vi "Read ADU Packet.vi"(8 "error in":errorcluster, 10 "Network Protocol":refnum<class "Network Protocol.lvclass">, 11 "ASCII transmission data unit in":refnum<class "ASCII Data Unit.lvclass">) -> (0 "error out":errorcluster, 1 "modbus data unit":refnum<class "Modbus Data Unit.lvclass">, 2 "Network Protocol out":refnum<class "Network Protocol.lvclass">, 3 "ASCII transmission data unit out":refnum<class "ASCII Data Unit.lvclass">, 5 "PDU Valid?":bool)   [LabVIEW 2013, in "Modbus Library - Advance.lvlib" / "ASCII Data Unit.lvclass"]
uses:
  ASCII Data Unit.lvclass
  Modbus Data Unit/Modbus Data Unit.lvclass
  Network Protocol/Network Protocol.lvclass
  Network Protocol/Network Master/Serial/Serial Master.lvclass
  Network Protocol/Network Master/Serial/Serial Master.lvclass/Serial Master.ctl
  Network Protocol/Network Slave/Serial/Serial Slave.lvclass
  Network Protocol/Network Slave/Serial/Serial Slave.lvclass/Serial Slave.ctl
  Transmission Data Unit.lvclass/Transmission Data Unit.ctl
  Serial Interface/Serial Data Unit.lvclass/Serial Data Unit.ctl
  Modbus Data Unit/Modbus Data Unit.lvclass/Modbus Data Unit.ctl
  ASCII Data Unit.lvclass/ASCII Data Unit.ctl
  Serial Interface/Serial acquisition states.ctl
  <vilib>/ErrorRing/Error Ring.xnode
  Transmission Data Unit.lvclass
  Serial Interface/Serial Data Unit.lvclass
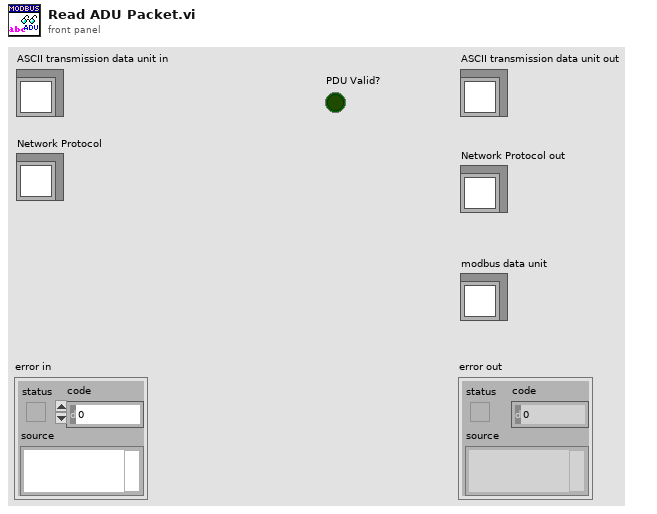
[diagram p1: front panel]
types:
  T1 = typedef "Modbus Library - Advance.lvlib/Serial Data Unit.lvclass/Serial acquisition states.ctl" = enum16{"Wait for frame", "Check for validity"}
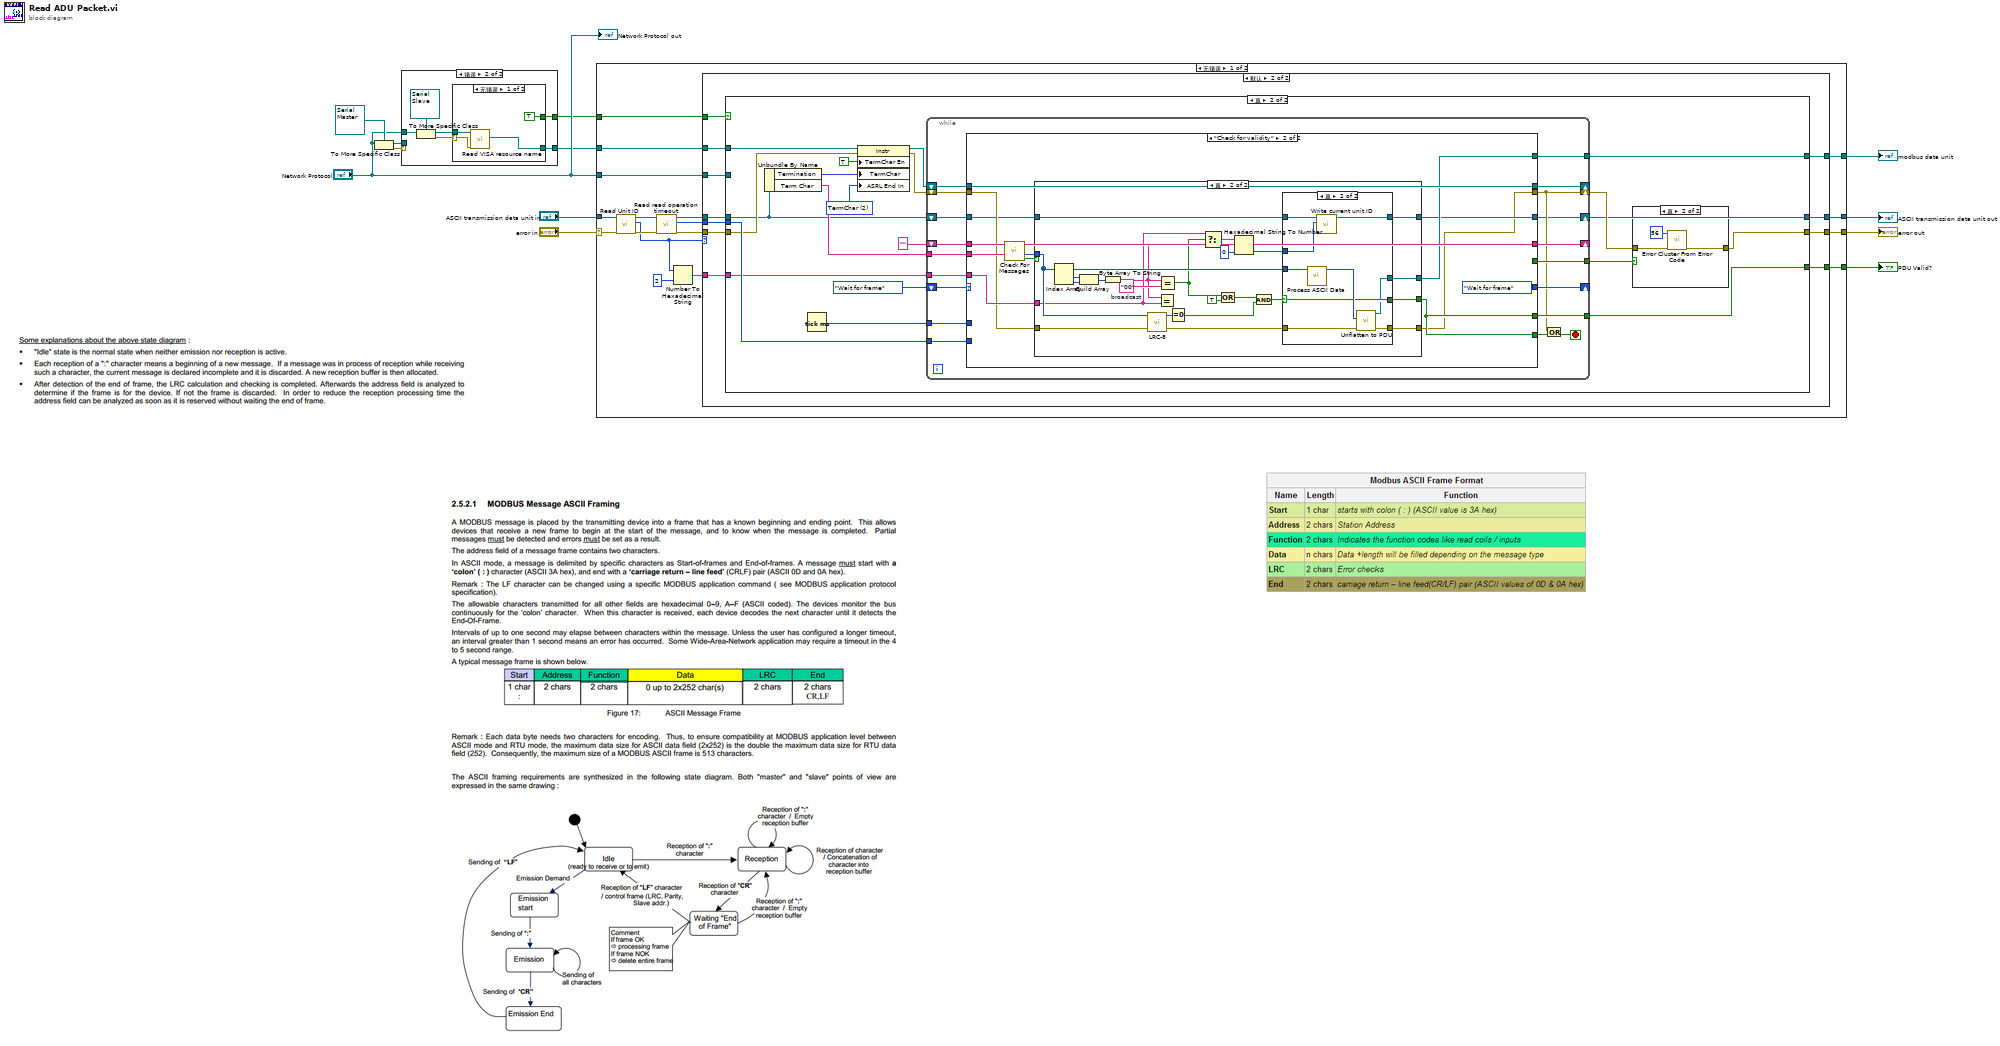
[diagram p0: block diagram]
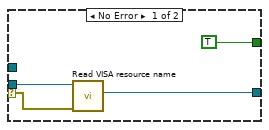
[diagram p2: hidden frame]
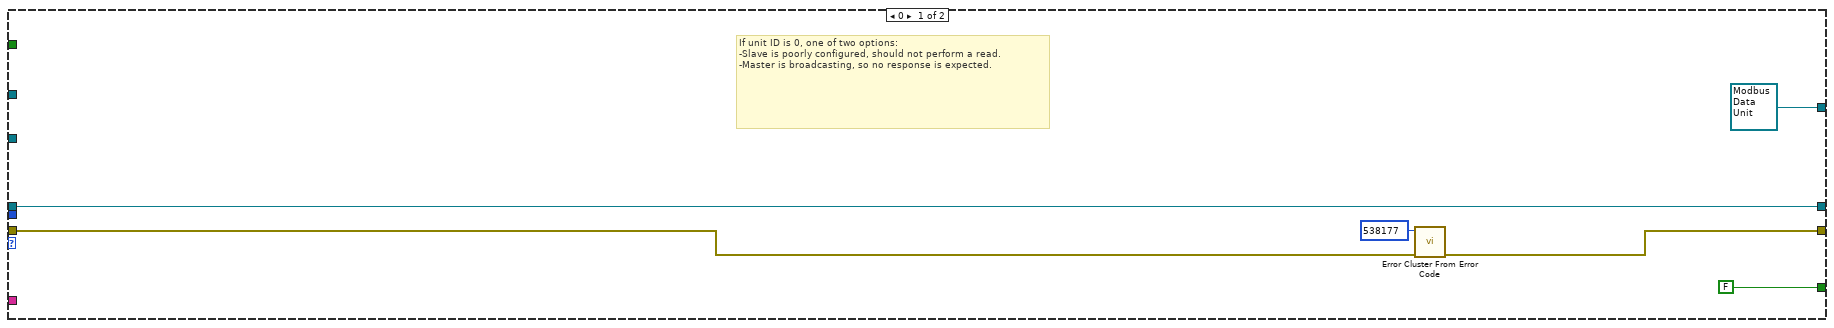
[diagram p4: hidden frame]
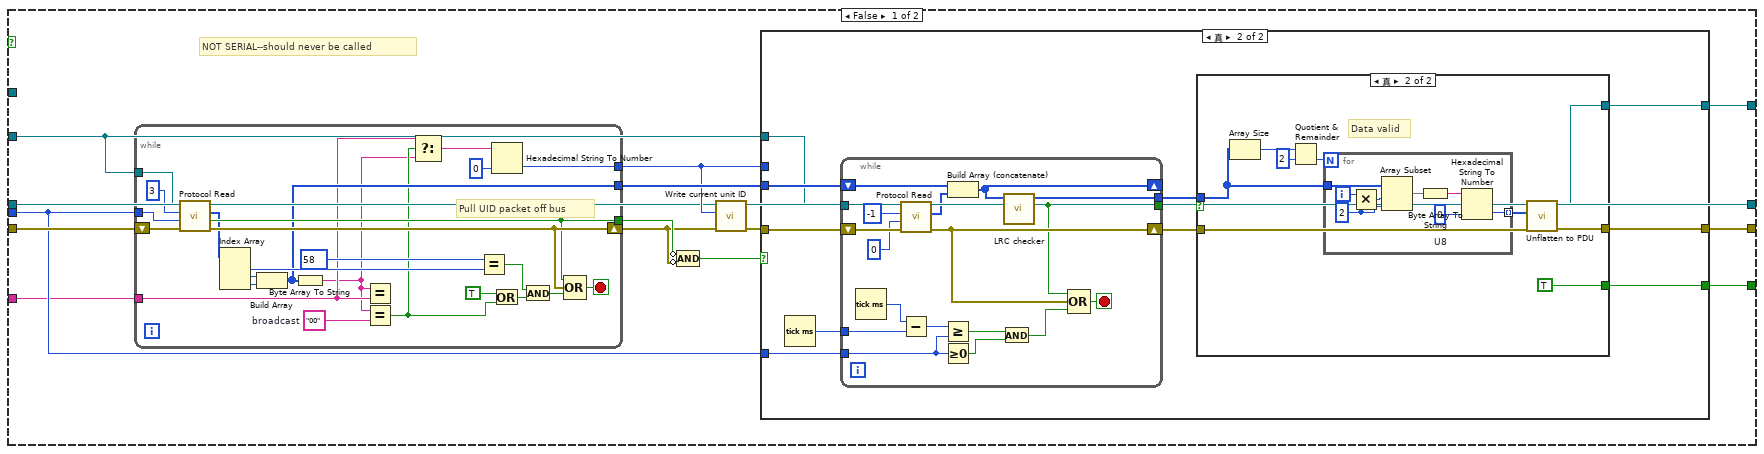
[diagram p5: hidden frame]
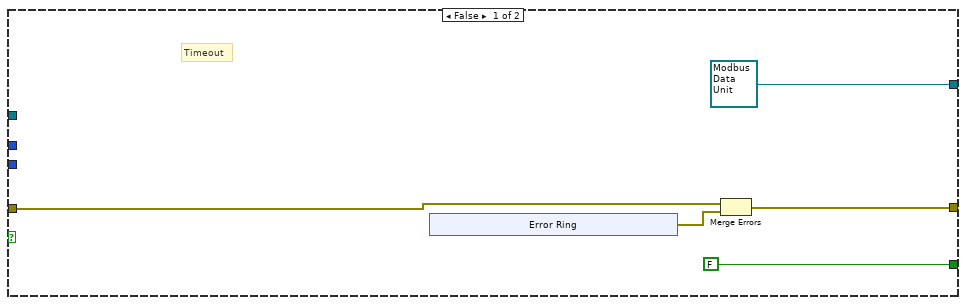
[diagram p6: hidden frame]
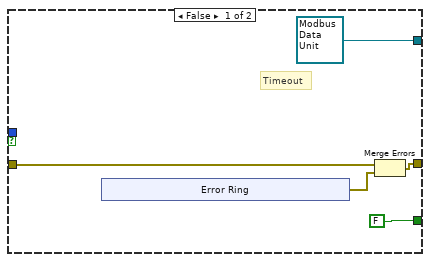
[diagram p7: hidden frame]
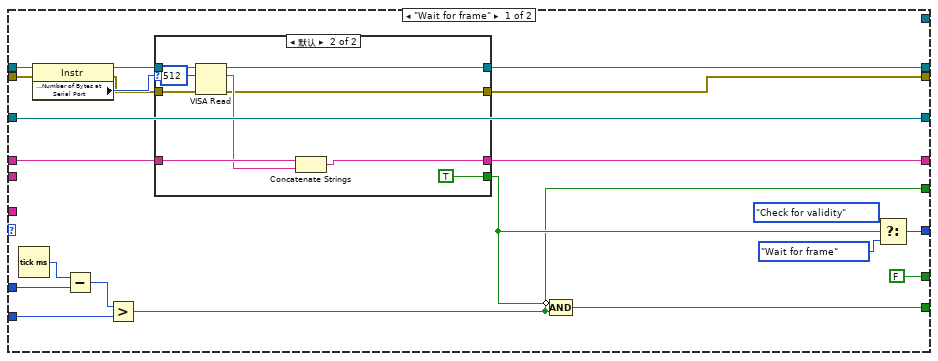
[diagram p9: hidden frame]
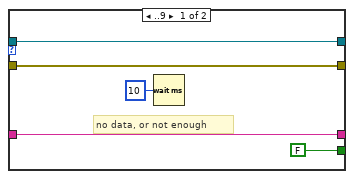
[diagram p10: hidden frame]
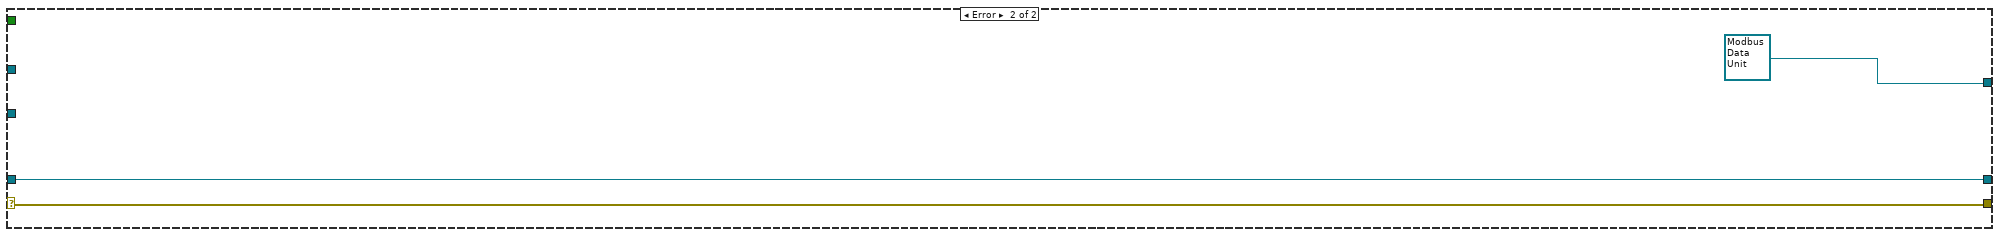
[diagram p13: hidden frame]
diagram:
  n1 = To More Specific Class(target class=refnum<class "Serial Master.lvclass"> refnum ("Serial Master"), reference="Network Protocol") -> (specific class reference=w3:refnum<class "Serial Master.lvclass">, error out=w6:errorcluster)  [unwired: 1 in]
  n2 = case shown="错误" w6 {
    selector: w6 -> [w14 _]
    tunnel: "Network Protocol" -> [_ w22]
    tunnel: [TRUE w19] -> w4
    tunnel: w3 -> [w15 _]
    tunnel: [w13 w17] -> w2
    frame No Error {
      n3 = call "Read VISA resource name.vi"("error in (no error)"=w14, "Serial Master in"=w15) -> ("VISA resource name"=w13:refnum<visa-resource-name>)  [unwired: 7 in, 2 out]
    }
    frame Error {
      n4 = To More Specific Class(target class=refnum<class "Serial Slave.lvclass"> refnum ("Serial Slave"), reference=w22) -> (specific class reference=w18:refnum<class "Serial Slave.lvclass">, error out=w20:errorcluster)  [unwired: 1 in]
      n5 = case shown="无错误" w20 {
        selector: w20 -> [w24 _]
        tunnel: [TRUE _] -> w19
        tunnel: w18 -> [w25 _]
        tunnel: [w23 _] -> w17
        frame No Error {
          n6 = call "Read VISA resource name.vi"("error in (no error)"=w24, "Serial Slave in"=w25) -> ("VISA resource name"=w23:refnum<visa-resource-name>)  [unwired: 7 in, 2 out]
        }
        frame Error {
        }
      }
    }
  }
  n7 = case shown="无错误" "error in" {
    selector: "error in" -> [w39 w295]
    tunnel: [w43 w295] -> w9
    tunnel: "ASCII transmission data unit in" -> [w29 w293]
    tunnel: "Network Protocol" -> [w41 _]
    tunnel: [w42 refnum<class "Modbus Data Unit.lvclass"> refnum ("modbus data unit")] -> w10
    tunnel: [w35 _] -> w8
    tunnel: w4 -> [w34 _]
    tunnel: w2 -> [w30 _]
    tunnel: [w27 w293] -> w1
    frame No Error {
      n8 = call "Read Unit ID.vi"("error in"=w39, "transmission data unit in"=w29) -> ("error out"=w38:errorcluster, "unit ID"=w32:u8, "transmission data unit out"=w40:refnum<class "ASCII Data Unit.lvclass">)  [unwired: 7 in]
      n9 = call "Read read operation timeout.vi"("error in (no error)"=w38, "transmission data unit in"=w40) -> ("error out"=w37:errorcluster, "read operation timeout"=w36:i32, "transmission data unit out"=w28:refnum<class "ASCII Data Unit.lvclass">)  [unwired: 7 in]
      n10 = Number To Hexadecimal String(1:i16 2 ("width (-)"), 2:w32) -> (0:w31:string)
      n11 = case shown="默认" w32 {
        tunnel: w37 -> [w49 w56]
        tunnel: [w46 w60] -> w43
        tunnel: [refnum<class "Modbus Data Unit.lvclass"> refnum ("modbus data unit out") w59] -> w42
        tunnel: w41 -> [_ w55]
        tunnel: w36 -> [_ w58]
        tunnel: [FALSE w57] -> w35
        tunnel: w34 -> [_ w54]
        tunnel: w31 -> [_ w53]
        tunnel: w30 -> [_ w52]
        tunnel: w28 -> [w44 w51]
        tunnel: [w44 w50] -> w27
        frame 0 {
          # "If unit ID is 0, one of two options:\n-Slave is poorly configured, should not perform a read.\n-Master is broadcasting, so no response is expected."
          n12 = call <vilib>:"Error Cluster From Error Code.vi"("error in (no error)"=w49, "error code (0)"=538177) -> ("error out"=w46:errorcluster)  [unwired: 7 in]
        }
        frame Default {
          n13 = case shown="真" w54 {
            tunnel: w56 -> [w75 w173]
            tunnel: [w72 w167] -> w60
            tunnel: [w71 w166] -> w59
            tunnel: w55 -> [w70 _]
            tunnel: w58 -> [w68 w174]
            tunnel: [w67 w172] -> w57
            tunnel: w53 -> [w66 w170]
            tunnel: w52 -> [_ w181]
            tunnel: w51 -> [w63 w165]
            tunnel: [w62 w164] -> w50
            frame False {
              # "NOT SERIAL--should never be called"
              n14 = while {
                shift-right: [w160] -> w65
                shift-left: w75 -> [w163]
                tunnel: w68 -> [w158]
                tunnel: [w156] -> w74
                tunnel: [w149] -> w69
                tunnel: w70 -> [w162]
                tunnel: w66 -> [w143]
                tunnel: [w140] -> w64
                stop <- w161 stop-if-true
                w147 = "00"  # broadcast
                # "Pull UID packet off bus"
                n15 = call-dynamic "Protocol Read.vi"("error in"=w163, "timeout"=w158, "bytes to read"=3, "protocol layer in"=w162) -> ("error out"=w160:errorcluster, "timed out?"=w156:bool, "data"=w155:u8[])  [unwired: 4 in, 1 out]
                n16 = Index Array(array=w155) -> (element #1=w153:u8, element #2=w151:u8, element #3=w150:u8)  [unwired: 3 in]
                n17 = Build Array(w151, w150) -> (w149:u8[])
                n18 = Byte Array To String(unsigned byte array=w149) -> (string=w142:string)
                n19 = Equal?(x=w142, y=w143) -> ()  [unwired: 1 out]
                n20 = Equal?(x=w142, y=w147) -> (x = y?=w144:bool)
                n21 = Select(t=w143, s=w144, f=w142) -> (s? t:f=w141:string)
                n22 = Equal?(x=u8 58 ("y"), y=w153) -> (x = y?=w152:bool)
                n23 = Hexadecimal String To Number(string=w141, default (0uL)=u8 0 ("默认(0 U32)")) -> (number=w140:u8)  [unwired: 1 in, 1 out]
                n24 = Or(x=TRUE, y=w144) -> (x .or. y?=w148:bool)
                n25 = And(x=w152, y=w148) -> (x .and. y?=w157:bool)
                n26 = Compound Arithmetic op=OR(w156, w160, w157) -> (w161:bool)
              }
              n27 = Compound Arithmetic op=AND(invert w74, invert w65) -> (w73:bool)
              n28 = call "Write current unit ID.vi"("error in (no error)"=w65, "request unit ID"=w64, "Serial Data Unit in"=w63) -> ("error out"=w61:errorcluster, "Serial Data Unit out"=w62:refnum<class "ASCII Data Unit.lvclass">)  [unwired: 7 in]
              n29 = case shown="真" w73 {
                tunnel: w61 -> [w78 w95]
                tunnel: [w79 w87] -> w72
                tunnel: [refnum<class "Modbus Data Unit.lvclass"> refnum ("modbus data unit out") w88] -> w71
                tunnel: w70 -> [_ w91]
                tunnel: w69 -> [_ w92]
                tunnel: w68 -> [_ w93]
                tunnel: [FALSE w85] -> w67
                tunnel: w64 -> [_ _]
                frame False {
                  # "Timeout"
                  n30 = xnode "Error Ring"() -> ("错误输出"=w80:errorcluster)
                  n31 = Merge Errors(w78, w80) -> (w79:errorcluster)
                }
                frame True {
                  n32 = Tick Count (ms)() -> (millisecond timer value=w94:u32)
                  n33 = while {
                    shift-right: [w125] -> w89
                    shift-left: w95 -> [w131]
                    tunnel: w94 -> [w139]
                    tunnel: w93 -> [w136]
                    shift-right: [w124] -> _
                    shift-left: w92 -> [w127]
                    tunnel: w91 -> [w130]
                    tunnel: [w122] -> w90
                    tunnel: [w123] -> w86
                    stop <- w133 stop-if-true
                    n34 = Tick Count (ms)() -> (millisecond timer value=w138:u32)
                    n35 = call-dynamic "Protocol Read.vi"("error in"=w131, "timeout"=0, "bytes to read"=-1, "protocol layer in"=w130) -> ("error out"=w125:errorcluster, "data"=w126:u8[])  [unwired: 4 in, 2 out]
                    n36 = Subtract(x=w138, y=w139) -> (x-y=w137:u32)
                    n37 = Greater Or Equal?(x=w137, y=w136) -> (x >= y?=w134:bool)
                    n38 = Greater Or Equal To 0?(x=w136) -> (x >= 0?=w135:bool)
                    n39 = Build Array (concatenate)(w127, w126) -> (w124:u8[])
                    n40 = And(x=w134, y=w135) -> (x .and. y?=w132:bool)
                    n41 = call "LRC checker.vi"("Data In"=w124) -> ("Valid?"=w122:bool, "Function Data Out"=w123:u8[])  [unwired: 9 in]
                    n42 = Compound Arithmetic op=OR(w122, w125, w132) -> (w133:bool)
                  }
                  n43 = case shown="真" w90 {
                    tunnel: w89 -> [w98 w111]
                    tunnel: [refnum<class "Modbus Data Unit.lvclass"> refnum ("modbus data unit") w112] -> w88
                    tunnel: [w97 w113] -> w87
                    tunnel: w86 -> [_ w106]
                    tunnel: [FALSE TRUE] -> w85
                    frame False {
                      # "Timeout"
                      n44 = xnode "Error Ring"() -> ("错误输出"=w99:errorcluster)
                      n45 = Merge Errors(w98, w99) -> (w97:errorcluster)
                    }
                    frame True {
                      # "Data valid"
                      n46 = Array Size(array=w106) -> (size(s)=w110:i32)
                      n47 = Quotient & Remainder(x=w110, y=2) -> (floor(x/y)=w108:i32)  [unwired: 1 out]
                      n48 = for {
                        N: w108 -> [_]
                        tunnel: w106 -> [w121]
                        tunnel: [w114] -> w107 mode=indexing
                        i -> [w120]
                        w115 = u8 0  # U8
                        w119 = 2 ("length")
                        n49 = Multiply(x=w120, y=w119) -> (x*y=w118:i32)
                        n50 = Array Subset(array=w121, index=w118, length=w119) -> (w117:u8[])
                        n51 = Byte Array To String(unsigned byte array=w117) -> (string=w116:string)
                        n52 = Hexadecimal String To Number(string=w116, default (0uL)=w115) -> (number=w114:u8)  [unwired: 2 out]
                      }
                      n53 = call "Unflatten to PDU.vi"("error in"=w111, "modbus data unit data"=w107) -> ("error out"=w113:errorcluster, "modbus data unit out"=w112:refnum<class "Modbus Data Unit.lvclass">)  [unwired: 8 in]
                    }
                  }
                }
              }
            }
            frame True {
              w182 = u16 2 items=["None", "Last Bit", "TermChar"] ("Serial Settings:End Mode for Reads")
              n54 = Unbundle By Name(w165) -> ("Termination"=w180:u8, "Term Char"=w171:string)
              n55 = Tick Count (ms)() -> (millisecond timer value=w175:u32)
              n56 = property class="Instr"(reference=w181, error in=w173, "TermChar En"=TRUE ("Message Based Settings:Termination Character Enable"), "TermChar"=w180, "ASRL End In"=w182) -> (reference out=w178:refnum<visa-resource-name>, error out=w177:errorcluster)
              n57 = while {
                shift-right: [w205] -> _
                shift-left: Serial_acquisition_states."Wait for frame" ("Serial Acquisition States") -> [w206]
                shift-right: [w190] -> w168
                shift-left: w177 -> [w203]
                shift-right: [w197] -> _
                shift-left: w178 -> [w204]
                shift-right: [w201] -> _
                shift-left: "" -> [w202]
                tunnel: w175 -> [w200]
                tunnel: w174 -> [w199]
                tunnel: [w196] -> w172
                tunnel: w171 -> [w195]
                tunnel: w170 -> [w194]
                tunnel: [w193] -> w169
                tunnel: [w192] -> w166
                shift-right: [w188] -> w164
                shift-left: w165 -> [w189]
                stop <- w191 stop-if-true
                n58 = case shown="\"Check for validity\"" w206 {
                  tunnel: [w227 Serial_acquisition_states."Wait for frame" ("Serial Acquisition States")] -> w205
                  tunnel: w204 -> [w222 w254]
                  tunnel: w203 -> [w221 w245]
                  tunnel: w202 -> [w220 w253]
                  tunnel: [w219 w251] -> w201
                  tunnel: w200 -> [w217 _]
                  tunnel: w199 -> [w215 _]
                  tunnel: [w210 w247] -> w198
                  tunnel: [w212 w242] -> w190
                  tunnel: [w211 w254] -> w197
                  tunnel: [FALSE w247] -> w196
                  tunnel: w195 -> [_ w252]
                  tunnel: w194 -> [_ w249]
                  tunnel: [w208 _] -> w193
                  tunnel: [_ w246] -> w192
                  tunnel: w189 -> [w207 w244]
                  tunnel: [w207 w243] -> w188
                  frame "Wait for frame" {
                    n59 = Tick Count (ms)() -> (millisecond timer value=w218:u32)
                    n60 = property class="Instr"(reference=w222, error in=w221) -> (reference out=w224:refnum<visa-resource-name>, error out=w213:errorcluster, "Serial Settings:Number of Bytes at Serial Port"=w223:u32)
                    n61 = Subtract(x=w218, y=w217) -> (x-y=w216:u32)
                    n62 = Greater?(x=w216, y=w215) -> (0:w208:bool)
                    n63 = case shown="默认" w223 {
                      tunnel: w224 -> [w228 w241]
                      tunnel: w220 -> [w231 w240]
                      tunnel: [w231 w238] -> w219
                      tunnel: [FALSE TRUE] -> w214
                      tunnel: w213 -> [w229 w236]
                      tunnel: [w229 w235] -> w212
                      tunnel: [w228 w234] -> w211
                      frame ..9 {
                        # "no data, or not enough"
                        n64 = Wait (ms)(milliseconds to wait=u32 10) -> ()  [unwired: 1 out]
                      }
                      frame Default {
                        n65 = VISA Read(VISA resource name=w241, byte count=u32 512, error in (no error)=w236) -> (VISA resource name out=w234:refnum<visa-resource-name>, read buffer=w239:string, error out=w235:errorcluster)  [unwired: 1 out]
                        n66 = Concatenate Strings(w240, w239) -> (w238:string)
                      }
                    }
                    n67 = Compound Arithmetic op=AND(invert w214, w208) -> (w210:bool)
                    n68 = Select(t=Serial_acquisition_states."Check for validity" ("Serial Acquisition States"), s=w214, f=Serial_acquisition_states."Wait for frame" ("Serial Acquisition States")) -> (s? t:f=w227:T1)
                  }
                  frame "Check for validity" {
                    n69 = call "Check For Messages.vi"("Term Char"=w252, "Input String"=w253) -> ("found?"=w248:bool, "data"=w250:u8[], "Remaining String"=w251:string)  [unwired: 7 in]
                    n70 = case shown="真" w248 {
                      selector: w248 -> [w258 _]
                      tunnel: w250 -> [_ w272]
                      tunnel: w249 -> [_ w266]
                      tunnel: w245 -> [w257 w271]
                      tunnel: [w258 w270] -> w247
                      tunnel: [_ w269] -> w246
                      tunnel: [w257 w268] -> w242
                      tunnel: w244 -> [w256 w261]
                      tunnel: [w256 w259] -> w243
                      frame False {
                      }
                      frame True {
                        w278 = "00"  # broadcast
                        n71 = Index Array(array=w272) -> (element #1=w276:u8, element #2=w277:u8)  [unwired: 2 in]
                        n72 = Build Array(w276, w277) -> (w275:u8[])
                        n73 = Byte Array To String(unsigned byte array=w275) -> (string=w265:string)
                        n74 = call "LRC-8.vi"("data"=w272) -> ("LRC-8"=w279:u8)  [unwired: 10 in]
                        n75 = Equal?(x=w265, y=w266) -> ()  [unwired: 1 out]
                        n76 = Equal?(x=w265, y=w278) -> (x = y?=w267:bool)
                        n77 = Equal To 0?(x=w279) -> (x = 0?=w280:bool)
                        n78 = Select(t=w266, s=w267, f=w265) -> (s? t:f=w263:string)
                        n79 = Or(x=w267, y=TRUE) -> (x .or. y?=w274:bool)
                        n80 = Hexadecimal String To Number(string=w263, default (0uL)=u8 0 ("默认(0 U32)")) -> (number=w260:u8)  [unwired: 1 in, 1 out]
                        n81 = Compound Arithmetic op=AND(w274, w280) -> (w273:bool)
                        n82 = case shown="真" w273 {
                          selector: w273 -> [w283 w289]
                          tunnel: w272 -> [_ w292]
                          tunnel: w271 -> [w282 w291]
                          tunnel: [w283 w289] -> w270
                          tunnel: [_ w288] -> w269
                          tunnel: [w282 w287] -> w268
                          tunnel: w261 -> [w281 w286]
                          tunnel: w260 -> [_ w285]
                          tunnel: [w281 w284] -> w259
                          frame False {
                          }
                          frame True {
                            n83 = call "Process ASCII Data.vi"("data"=w292) -> ("pdu"=w290:u8[])  [unwired: 10 in]
                            n84 = call "Write current unit ID.vi"("request unit ID"=w285, "Serial Data Unit in"=w286) -> ("Serial Data Unit out"=w284:refnum<class "ASCII Data Unit.lvclass">)  [unwired: 8 in, 1 out]
                            n85 = call "Unflatten to PDU.vi"("error in"=w291, "modbus data unit data"=w290) -> ("error out"=w287:errorcluster, "modbus data unit out"=w288:refnum<class "Modbus Data Unit.lvclass">)  [unwired: 8 in]
                          }
                        }
                      }
                    }
                  }
                }
                n86 = Or(x=w190, y=w198) -> (x .or. y?=w191:bool)
              }
              n87 = case shown="真" w169 {
                tunnel: w168 -> [w184 w187]
                tunnel: [w184 w185] -> w167
                frame False {
                }
                frame True {
                  n88 = call <vilib>:"Error Cluster From Error Code.vi"("error in (no error)"=w187, "error code (0)"=56) -> ("error out"=w185:errorcluster)  [unwired: 7 in]
                }
              }
            }
          }
        }
      }
    }
    frame Error {
    }
  }
  "modbus data unit" <- w10
  "error out" <- w9
  "PDU Valid?" <- w8
  "ASCII transmission data unit out" <- w1
  "Network Protocol out" <- "Network Protocol"
